vi "set_alignment_mode.vi"(8 "error in (no error)":errorcluster, 10 "alignment mode?":bool, 11 "LightSourceAN191011Chameleon in":refnum<class "LightSourceAN191011Chameleon.lvclass">) -> (0 "error out":errorcluster, 3 "LightSourceAN191011Chameleon out":refnum<class "LightSourceAN191011Chameleon.lvclass">)   [LabVIEW 2011, in "LightSourceAN191011Chameleon.lvclass"]
uses:
  LightSourceAN191011Chameleon.lvclass
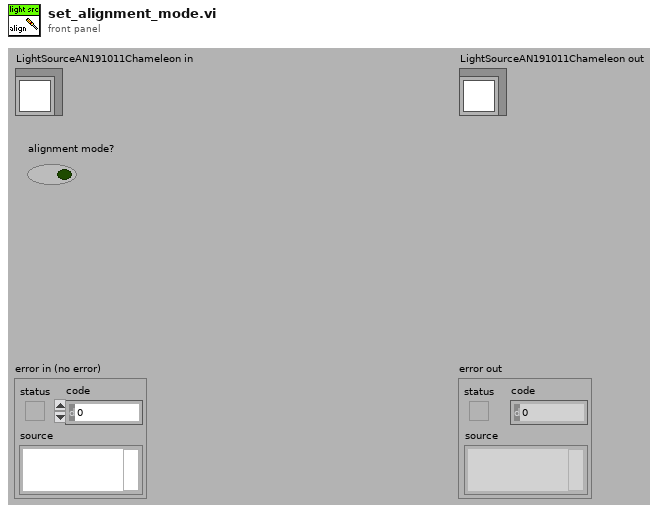
[diagram p1: front panel]
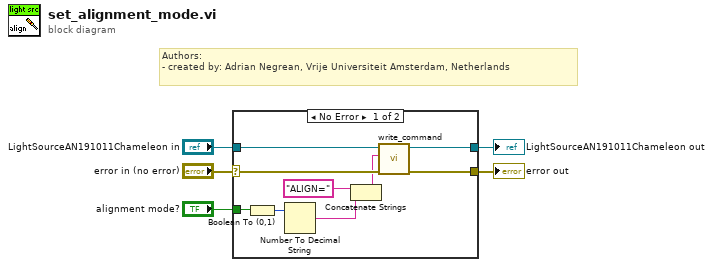
[diagram p0: block diagram]
diagram:
  # "Authors: \n- created by: Adrian Negrean, Vrije Universiteit Amsterdam, Netherlands"
  n1 = case shown="No Error" "error in (no error)" {
    selector: "error in (no error)" -> [w12 w16]
    tunnel: [w11 w16] -> w4
    tunnel: [w13 w15] -> w2
    tunnel: "LightSourceAN191011Chameleon in" -> [w14 w15]
    tunnel: "alignment mode?" -> [w7 _]
    frame No Error {
      n2 = Boolean To (0,1)(Boolean=w7) -> (0, 1=w10:i16)
      n3 = Number To Decimal String(number=w10) -> (decimal integer string=w8:string)  [unwired: 1 in]
      n4 = Concatenate Strings("ALIGN=" ("string"), w8) -> (w6:string)
      n5 = call-dynamic "write_command.vi"("error in (no error)"=w12, "string to write"=w6, "LightSourceAN191011Chameleon in"=w14) -> ("error out"=w11:errorcluster, "LightSourceAN191011Chameleon out"=w13:refnum<class "LightSourceAN191011Chameleon.lvclass">)  [unwired: 6 in, 1 out]
    }
    frame Error {
    }
  }
  "error out" <- w4
  "LightSourceAN191011Chameleon out" <- w2
